vi "Initialize.vi"(8 "error in (no error)":errorcluster, 10 "Input":T1, 11 "Driver in":refnum<class "Driver.lvclass">) -> (0 "error out":errorcluster, 3 "Driver out":refnum<class "Driver.lvclass">)   [LabVIEW 2023, in "Driver.lvlib" / "Driver.lvclass"]
uses:
  Driver.lvclass
  Driver.lvclass/Driver.ctl
  <vilib>/Instr/_visa.llb/VISA Configure Serial Port (Instr).vi
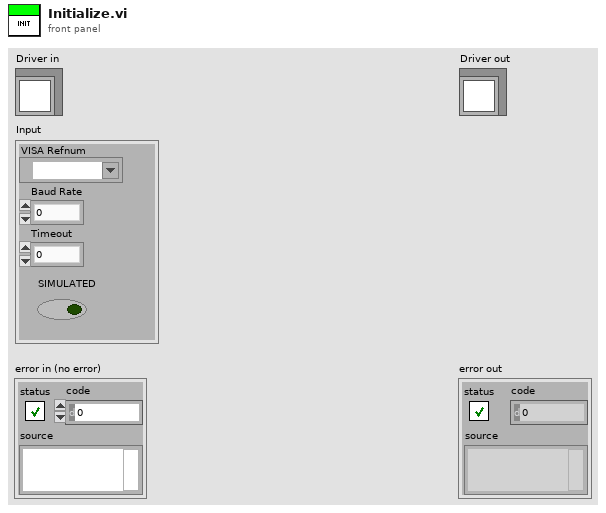
[diagram p1: front panel]
types:
  T1 = cluster{"VISA Refnum":refnum<visa-resource-name>, "Baud Rate":u32, "Timeout":u32, "SIMULATED":bool}
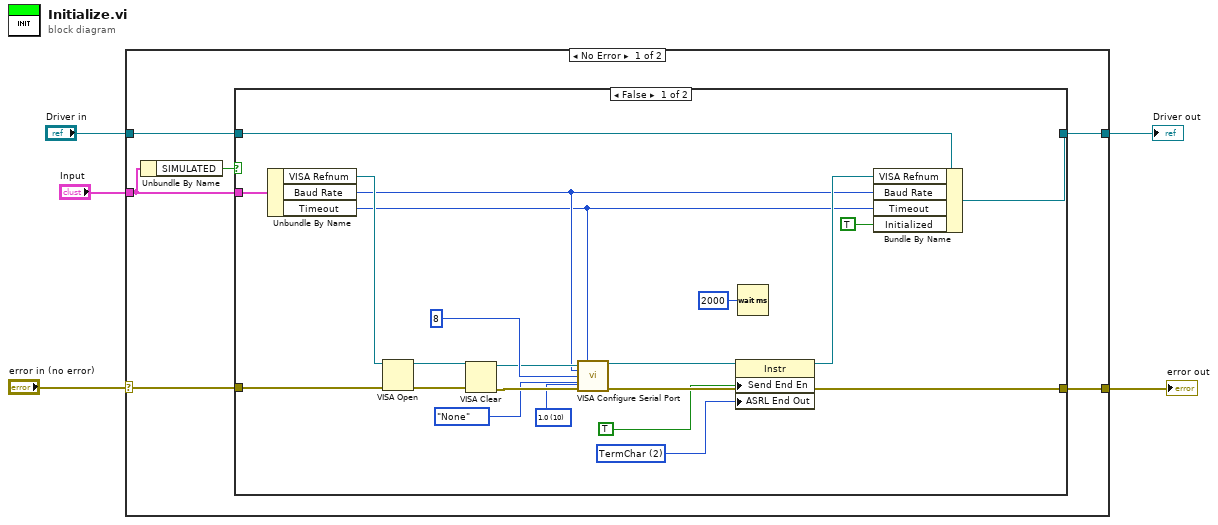
[diagram p0: block diagram]
diagram:
  n1 = case shown="No Error" "error in (no error)" {
    selector: "error in (no error)" -> [w11 w37]
    tunnel: [w10 w37] -> w4
    tunnel: [w8 w36] -> w2
    tunnel: "Driver in" -> [w9 w36]
    tunnel: "Input" -> [w7 _]
    frame No Error {
      n2 = Unbundle By Name(w7) -> ("SIMULATED"=w6:bool)
      n3 = case shown="False" w6 {
        tunnel: w11 -> [w33 w34]
        tunnel: [w21 w34] -> w10
        tunnel: w9 -> [w20 w35]
        tunnel: [w19 w35] -> w8
        tunnel: w7 -> [w12 _]
        frame False {
          w25 = u16 2 items=["None", "Last Bit", "TermChar", "Break"] ("Serial Settings:End Mode for Writes")
          w26 = u16 10 items=["1.0"=10, "1.5"=15, "2.0"=20] ("stop bits (10: 1 bit)")
          n4 = Unbundle By Name(w12) -> ("VISA Refnum"=w32:refnum<visa-resource-name>, "Baud Rate"=w17:u32, "Timeout"=w16:u32)
          n5 = VISA Open(error in (no error)=w33, VISA resource name=w32) -> (VISA resource name=w15:refnum<visa-resource-name>, error out=w31:errorcluster)  [unwired: 3 in]
          n6 = VISA Clear(VISA resource name=w15, error in (no error)=w31) -> (VISA resource name out=w27:refnum<visa-resource-name>, error out=w30:errorcluster)
          n7 = call-poly "VISA Configure Serial Port"("VISA resource name"=w27, "timeout (10sec)"=w16, "baud rate (9600)"=w17, "data bits (8)"=u16 8, "parity (0:none)"=enum16{"None", "Odd", "Even", "Mark", "Space"}."None", "error in (no error)"=w30, "stop bits (10: 1 bit)"=w26) -> ("VISA resource name out"=w24:refnum<visa-resource-name>, "error out"=w23:errorcluster)  [unwired: 7 in]
          n8 = property class="Instr"(reference=w24, error in=w23, "Send End En"=TRUE ("Message Based Settings:Send End Enable"), "ASRL End Out"=w25) -> (reference out=w18:refnum<visa-resource-name>, error out=w21:errorcluster)
          n9 = Wait (ms)(milliseconds to wait=u32 2000) -> ()  [unwired: 1 out]
          n10 = Bundle By Name(cluster=w20, "VISA Refnum"=w18, "Baud Rate"=w17, "Timeout"=w16, "Initialized"=TRUE) -> (w19:refnum<class "Driver.lvclass">)
        }
        frame True {
        }
      }
    }
    frame Error {
    }
  }
  "error out" <- w4
  "Driver out" <- w2
